vi "General Histogram.vi"(0 "X":dbl[](array[numeric]) format="%0.2f", 5 "Bins":T2(array[cluster]) {"upper" format="%0.2f"; "lower" format="%0.2f"}, 7 "max":dbl format="%0.2f", 9 "min":dbl format="%0.2f", 11 "# bins":i32, 12 "inclusion":enum32{"lower", "upper"}(ring)) -> (4 "Histogram Graph":T1(graph), 6 "Histogram":i32[](array[numeric]), 8 "Axis":dbl[](array[numeric]) format="%0.2f", 10 "# outside":cluster{"total":i32, "below":i32, "above":i32}, 15 "error":i32)   [LabVIEW 2020, in "NI_AALPro.lvlib"]
doc: "Finds the discrete histogram of the input sequence <B>X</B> based on the given bin specifications."
uses:
  <vilib>/Analysis/NI_AALPro.lvlib
  <resource>/lvanlys.dll
panel:
  # "General Histogram"
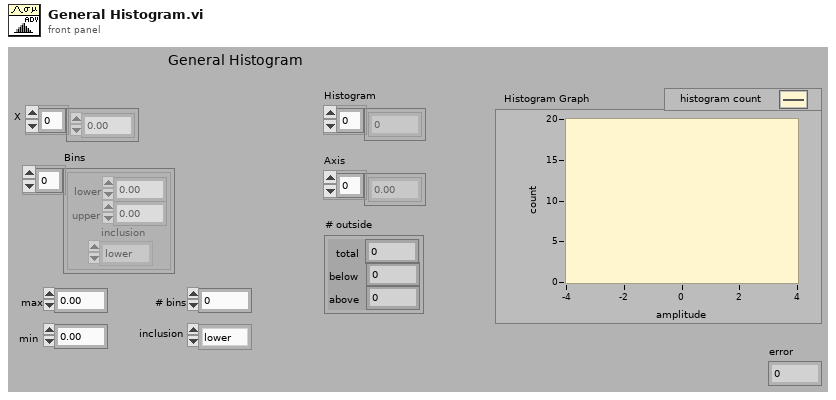
[diagram p1: front panel]
types:
  T1 = cluster{"X Values":dbl[], "Histogram: h(x)":i32[]}
  T2 = cluster{"lower":dbl, "upper":dbl, "inclusion":enum32{"lower", "upper", "both", "neither"}}[]
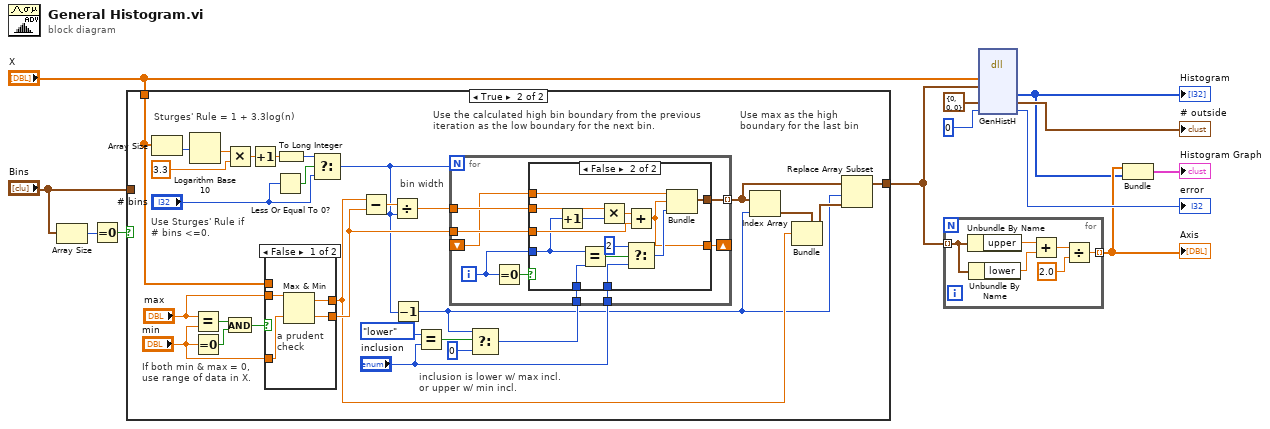
[diagram p0: block diagram]
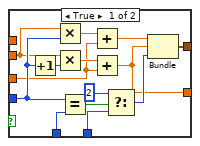
[diagram p3: hidden frame]
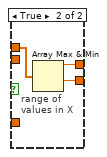
[diagram p4: hidden frame]
diagram:
  n1 = Array Size(array="Bins") -> (size(s)=w12:i32)
  n2 = Equal To 0?(x=w12) -> (x = 0?=w11:bool)
  n3 = case shown="True" w11 {
    tunnel: "Bins" -> [w13 _]
    tunnel: [w13 w19] -> w9
    tunnel: "X" -> [_ w37]
    frame False {
      # "Use the given bin specification"
    }
    frame True {
      # "Use max as the high boundary for the last bin"
      # "Use the calculated high bin boundary from the previous\niteration as the low boundary for the next bin."
      # "inclusion is lower w/ max incl.\nor upper w/ min incl."
      # "bin width"
      # "Use Sturges' Rule if\n# bins <=0."
      # "If both min & max = 0,\nuse range of data in X."
      # "Sturges' Rule = 1 + 3.3log(n)"
      n4 = Array Size(array=w37) -> (size(s)=w34:i32)
      n5 = Logarithm Base 10(1:w34) -> (0:w32:dbl)
      n6 = Equal?(x="max", y="min") -> (x = y?=w41:bool)
      n7 = Equal To 0?(x="min") -> (x = 0?=w42:bool)
      n8 = Multiply(x=w32, y=3.3) -> (x*y=w31:dbl)
      n9 = And(x=w41, y=w42) -> (x .and. y?=w40:bool)
      n10 = Increment(x=w31) -> (x+1=w30:dbl)
      n11 = case shown="False" w40 {
        tunnel: w37 -> [_ w85]
        tunnel: [w82 w84] -> w15
        tunnel: [w80 w83] -> w23
        tunnel: "max" -> [w81 _]
        tunnel: "min" -> [w79 _]
        frame False {
          # "a prudent\ncheck"
          n12 = Max & Min(x=w81, y=w79) -> (max(x,y)=w82:dbl, min(x,y)=w80:dbl)
        }
        frame True {
          # "range of \nvalues in X"
          n13 = Array Max & Min(array=w85) -> (max value=w84:dbl, min value=w83:dbl)  [unwired: 2 out]
        }
      }
      n14 = Less Or Equal To 0?(x="# bins") -> (x <= 0?=w36:bool)
      n15 = To Long Integer(number=w30) -> (32bit integer=w29:i32)
      n16 = Select(t=w29, s=w36, f="# bins") -> (s? t:f=w22:i32)
      n17 = Subtract(x=w15, y=w23) -> (x-y=w28:dbl)
      n18 = Divide(x=w28, y=w22) -> (x/y=w24:dbl)
      n19 = Decrement(x=w22) -> (x-1=w14:i32)
      n20 = Equal?(x=enum32{"lower", "upper"}."lower" ("inclusion"), y="inclusion") -> (x = y?=w27:bool)
      n21 = Select(t=w14, s=w27, f=0) -> (s? t:f=w25:i32)
      n22 = for {
        N: w22 -> [_]
        tunnel: w24 -> [w47]
        tunnel: "inclusion" -> [w49]
        tunnel: [w51] -> w18 mode=indexing
        tunnel: w23 -> [w50]
        tunnel: w25 -> [w48]
        shift-right: [w46] -> _
        shift-left: _ -> [w43]
        i -> [w45]
        n23 = Equal To 0?(x=w45) -> (x = 0?=w44:bool)
        n24 = case shown="False" w44 {
          tunnel: [w65 w78] -> w51
          tunnel: w50 -> [w52 w76]
          tunnel: w45 -> [w56 w67]
          tunnel: w49 -> [w61 w74]
          tunnel: w48 -> [w58 w71]
          tunnel: w47 -> [w54 w70]
          tunnel: [w57 w66] -> w46
          tunnel: w43 -> [_ w69]
          frame True {
            n25 = Increment(x=w56) -> (x+1=w55:i32)
            n26 = Multiply(x=w54, y=w56) -> (x*y=w64:dbl)
            n27 = Multiply(x=w54, y=w55) -> (x*y=w53:dbl)
            n28 = Equal?(x=w56, y=w58) -> (x = y?=w62:bool)
            n29 = Add(x=w64, y=w52) -> (x+y=w63:dbl)
            n30 = Add(x=w53, y=w52) -> (x+y=w57:dbl)
            n31 = Select(t=2, s=w62, f=w61) -> (s? t:f=w60:u32)
            n32 = Bundle(w63, w57, "inclusion"=w60) -> (w65:cluster{dbl, dbl, "inclusion":u32})  [unwired: 1 out]
          }
          frame False {
            n33 = Increment(x=w67) -> (x+1=w68:i32)
            n34 = Equal?(x=w67, y=w71) -> (x = y?=w75:bool)
            n35 = Multiply(x=w70, y=w68) -> (x*y=w77:dbl)
            n36 = Add(x=w77, y=w76) -> (x+y=w66:dbl)
            n37 = Select(t=2, s=w75, f=w74) -> (s? t:f=w73:u32)
            n38 = Bundle(w69, w66, "inclusion"=w73) -> (w78:cluster{dbl, dbl, "inclusion":u32})  [unwired: 1 out]
          }
        }
      }
      n39 = Index Array(array=w18, index=w14) -> (element=w17:cluster{dbl, dbl, "inclusion":u32})
      n40 = Bundle(cluster=w17, w15) -> (w16:cluster{dbl, dbl, "inclusion":u32})  [unwired: 2 out]
      n41 = Replace Array Subset(array=w18, new element=w16, index=w14) -> (w19:cluster{dbl, dbl, "inclusion":u32}[])
    }
  }
  n42 = for {
    tunnel: w9 -> [w91] mode=indexing
    tunnel: [w86] -> w4 mode=indexing
    n43 = Unbundle By Name(w91) -> ("upper"=w90:dbl)
    n44 = Unbundle By Name(w91) -> ("lower"=w89:dbl)
    n45 = Add(x=w90, y=w89) -> (x+y=w87:dbl)
    n46 = Divide(x=w87, y=2.0) -> (x/y=w86:dbl)
  }
  "Axis" <- w4
  n47 = dll-call lib="e:/builds/penguin/labview/branches/2020/dev/dist/resource/lvanlys.*" fn="GenHistH"("X"="X", "Bins"=w9, "# outside"=cluster{"total":i32, "below":i32, "above":i32} {"total"=0, "below"=0, "above"=0}, "output param"=0) -> ("Histogram"=w3:i32[], "# outside"=→"# outside":cluster{"total":i32, "below":i32, "above":i32}, "output param"=→"error":i32)  [unwired: 5 in, 4 out]
  "Histogram" <- w3
  n48 = Bundle(w4, "Histogram"=w3) -> (→"Histogram Graph":cluster{dbl[], "Histogram":i32[]})  [unwired: 1 out]
